vi "Autonomous Independent.vi"() -> ()   [LabVIEW 2014]
doc: "This VI is called when autonomous begins, and will automatically be terminated when autonomous ends. You can carry out timed or sensor driven robot movement independently without needing to return to the caller."
uses:
  Robot Global Data.vi
panel:
  in  "Autonomous Routine No.":u8
  # "Be sure to right-click and choose Data Operations>>Make Current Value default if you want to save the array values with the VI"
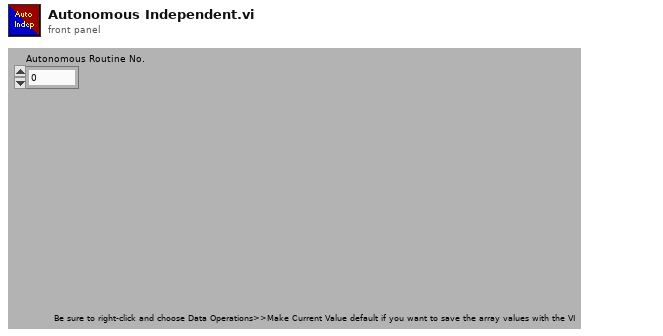
[diagram p1: front panel]
types:
  T1 = cluster{"X Position":dbl, "Y Position":dbl, "Angle":dbl}
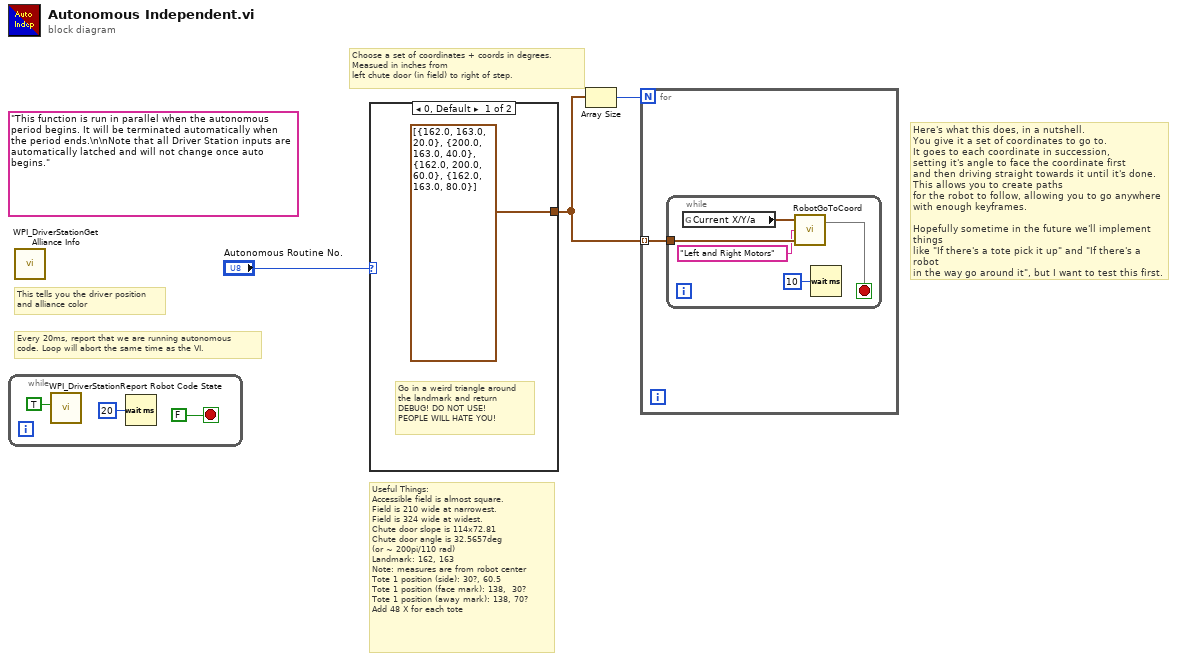
[diagram p0: block diagram]
diagram:
  (unwired) "This function is run in parallel when the autonomous period begins. It will be terminated automatically when the period ends.\n\nNote that all Driver Station inputs are automatically latched and will not change once auto begins."
  # "Useful Things:\nAccessible field is almost square.\nField is 210 wide at narrowest.\nField is 324 wide at widest. \nChute door slope is 114x72.81\nChute door angle is 32.5657deg\n(or ~ 200pi/110 rad) \nLandmark: 162, 163\nNote: measures are from robot center\nTote 1 position (side): 30?, 60.5 \nTote 1 position (face mark): 138,  30?\nTote 1 position (away mark): 138, 70? \nAdd 48 X for each tote"
  # "Choose a set of coordinates + coords in degrees.\nMeasued in inches from\nleft chute door (in field) to right of step."
  # "Here's what this does, in a nutshell.\nYou give it a set of coordinates to go to.\nIt goes to each coordinate in succession,\nsetting it's angle to face the coordinate first\nand then driving straight towards it until it's done.\nThis allows you to create paths\nfor the robot to follow, allowing you to go anywhere\nwith enough keyframes.\n\nHopefully sometime in the future we'll implement things\nlike \"If there's a tote pick it up\" and \"If there's a robot\nin the way go around it\", but I want to test this first."
  # "Every 20ms, report that we are running autonomous\ncode. Loop will abort the same time as the VI."
  # "This tells you the driver position\nand alliance color"
  n1 = while {
    stop <- FALSE stop-if-true
    n2 = call <vilib>:"WPI_DriverStationReport Robot Code State.vi"("Autonomous"=TRUE) -> ()  [unwired: 10 in, 1 out]
    n3 = Wait (ms)(milliseconds to wait=u32 20) -> ()  [unwired: 1 out]
  }
  n4 = call <vilib>:"WPI_DriverStationGet Alliance Info.vi"() -> ()  [unwired: 12 out]
  n5 = case shown="0, Default" "Autonomous Routine No." {
    tunnel: [cluster{dbl, dbl, dbl}[] [{162.0, 163.0, 20.0}, {200.0, 163.0, 40.0}, {162.0, 200.0, 60.0}, {162.0, 163.0, 80.0}] _] -> w1
    frame 0, Default {
      # "Go in a weird triangle around\nthe landmark and return\nDEBUG! DO NOT USE!\nPEOPLE WILL HATE YOU!"
    }
    frame 1 {
    }
  }
  n6 = Array Size(array=w1) -> (size(s)=w2:i32)
  n7 = for {
    N: w2 -> [_]
    tunnel: w1 -> [w8] mode=indexing
    n8 = while {
      tunnel: w8 -> [w10]
      stop <- w12 stop-if-true
      n9 = global read "Robot Global Data.vi" "Current X/Y/a"() -> (w11:T1)
      n10 = call "RobotGoToCoord.vi"("X/Y/a Target"=w10, "Drive Refnum"="Left and Right Motors" ("refnum name"), "X/Y/a Current"=w11) -> (0:w12)
      n11 = Wait (ms)(milliseconds to wait=u32 10) -> ()  [unwired: 1 out]
    }
  }
